vi "PFI-28000-Chan-28144_Get Excitation Tolerance.vi"(8 "error in (no error)":errorcluster, 11 "PFI-28000-Chan-28144 in":refnum<class "PFI-28000-Chan-28144.lvclass">) -> (0 "error out":errorcluster, 2 "Excitation Tolerance":dbl, 3 "PFI-28000-Chan-28144 out":refnum<class "PFI-28000-Chan-28144.lvclass">)   [LabVIEW 2017, in "PFI-28000-Chan-28144.lvclass"]
uses:
  PFI-28000-Chan-28144.lvclass
  C:/wc/07143 Precision Filters 28000 Support/Driver/source/Channel/PFI-28000-Channel.lvclass
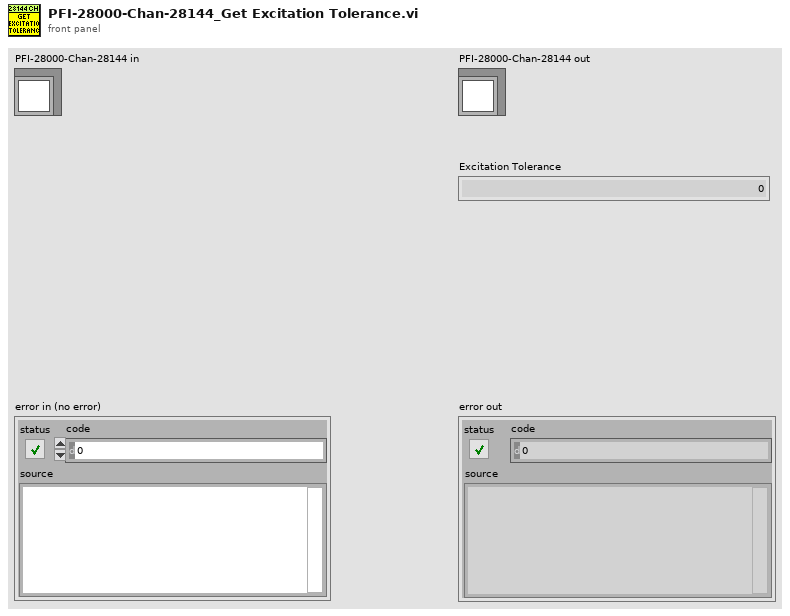
[diagram p1: front panel]
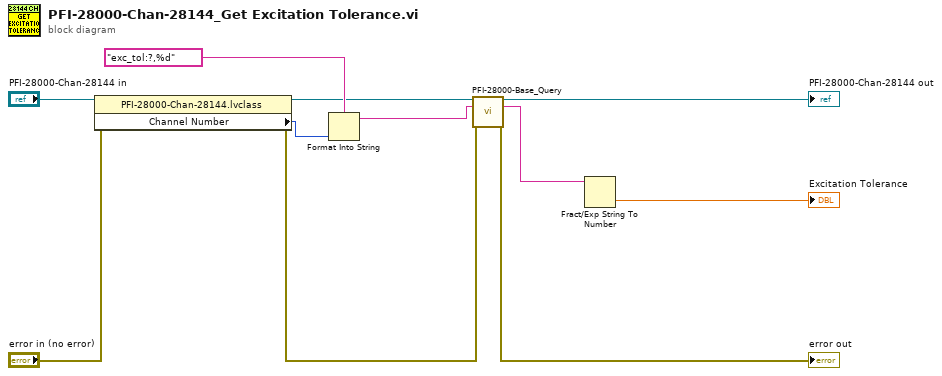
[diagram p0: block diagram]
diagram:
  n1 = property class="PFI-28000-Chan-28144.lvclass"(reference="PFI-28000-Chan-28144 in", error in="error in (no error)") -> (reference out=w7:refnum<class "PFI-28000-Chan-28144.lvclass">, error out=w4:errorcluster, "Channel Number"=w9:i32)
  n2 = Format Into String(format string="exc_tol:?,%d" ("empty string"), w9) -> (resulting string=w6:string)  [unwired: 2 in, 1 out]
  n3 = call-dynamic "PFI-28000-Base_Query.vi"("PFI-28000-Base in"=w7, "Command"=w6, "error in (no error)"=w4) -> ("PFI-28000-Base out"=→"PFI-28000-Chan-28144 out":refnum<class "PFI-28000-Chan-28144.lvclass">, "Response"=w2:string, "error out"=→"error out":errorcluster)  [unwired: 9 in, 1 out]
  n4 = Fract/Exp String To Number(string=w2) -> (number=→"Excitation Tolerance":dbl)  [unwired: 3 in, 1 out]
